vi "LEP_RV_MemorySettingsDlg.vi"(8 "error in (no error)":errorcluster, 10 "page sync rendezvous":T2, 11 "Close Event":refnum<user-event>) -> ()   [LabVIEW 2011]
doc: "This is the actual UI that the end user will see for configuring the build options."
uses:
  resource/dialog/PreferencesDialog/optionsFrame_EventData1.ctl
  resource/dialog/PreferencesDialog/optionsFrame_PageInitData.ctl
  <vilib>/Platform/EmbProject/Plugins/utilities/LEP_Utilities_GetSetProjectData_Variant.vi
panel:
  out "Tab Control":enum32{"Page 1", "Page 2"}(tab)
  in  "String":string
  in  "String 2":string
  in  "String 3":string
  in  "String 4":string
  in  "String 5":string
  in  "String 6":string
  in  "String 7":string
  in  "String 8":string
  in  "String 9":string
  in  "String 10":string
  in  "Boolean":bool
  in  "Boolean 2":bool
  in  "Boolean 3":bool
  in  "Boolean 4":bool
  in  "Boolean 5":bool
  in  "Boolean 6":bool
  in  "Boolean 7":bool
  in  "Boolean 8":bool
  in  "Boolean 9":bool
  in  "Boolean 10":bool
  in  "String 11":string
  in  "String 12":string
  in  "String 13":string
  in  "String 14":string
  in  "String 15":string
  in  "String 16":string
  in  "String 17":string
  in  "String 18":string
  in  "String 19":string
  in  "String 20":string
  in  "Boolean 11":bool
  in  "Boolean 12":bool
  in  "Boolean 13":bool
  in  "Boolean 14":bool
  in  "Boolean 15":bool
  in  "Boolean 16":bool
  in  "Boolean 17":bool
  in  "Boolean 18":bool
  in  "Boolean 19":bool
  in  "Boolean 20":bool
  in  "Ring 3":u16(ring) items=["<default>", "RAM1", "RAM2", "RAM3", "IRAM1", "IRAM2"]
  in  "Ring 2":u16(ring) items=["<default>", "RAM1", "RAM2", "RAM3", "IRAM1", "IRAM2"]
  in  "Ring":u16(ring) items=["<default>", "ROM1", "ROM2", "ROM3", "IROM1", "IROM2", "RAM1", "RAM2", "RAM3", "IRAM1", "IRAM2"]
  in  "Tree":string(tree)
  in  "Linker":path[](array[path])=[path ""]
  in  "Compiler":path[](array[path])=[path ""]
  out "Linker Flags":string
  out "Compiler Flags":string
  in  "ErrorFile":path
  in  "Extra LFlags":string
  in  "Extra CFlags":string
  in  "Debug Mode":u16(ring) items=["None", "Generate Debug Info", "On Chip", "On Chip (Release)"]
  in  "Generate C Function Calls":bool
  in  "Generate Integer Only":bool=TRUE
  in  "Show build warnings":bool
  in  "Build configuration":u16(ring) items=["Debug", "Release"]
  in  "Memory model":i32(ring) items=["Small", "Static"]
  in  "Use stack variables":bool
  in  "Generate serial only":bool
  in  "Generate guard code":bool
  in  "Page VI Init Data":T1
  in  "error msg format string":string="There was a problem applying the options from the %s category. The error message is \"%s.\""
  # "Build options"
  # "Debug options"
  # "Memory options"
  # "Run-time options"
  # "Read Only Memory Area"
  # "Default"
  # "Off-chip"
  # "Start"
  # "Size"
  # "Startup"
  # "ROM1:"
  # "ROM2:"
  # "ROM3:"
  # "On-chip"
  # "IROM1:"
  # "IROM2:"
  # "Read/Write Memory Area"
  # "Default"
  # "Off-chip"
  # "Start"
  # "Size"
  # "NoInit"
  # "RAM1:"
  # "RAM2:"
  # "RAM3:"
  # "On-chip"
  # "IRAM1:"
  # "IRAM2:"
  # "Memory Assignment"
  # "Code / Const:"
  # "Zero Initialized Data:"
  # "Other Data:"
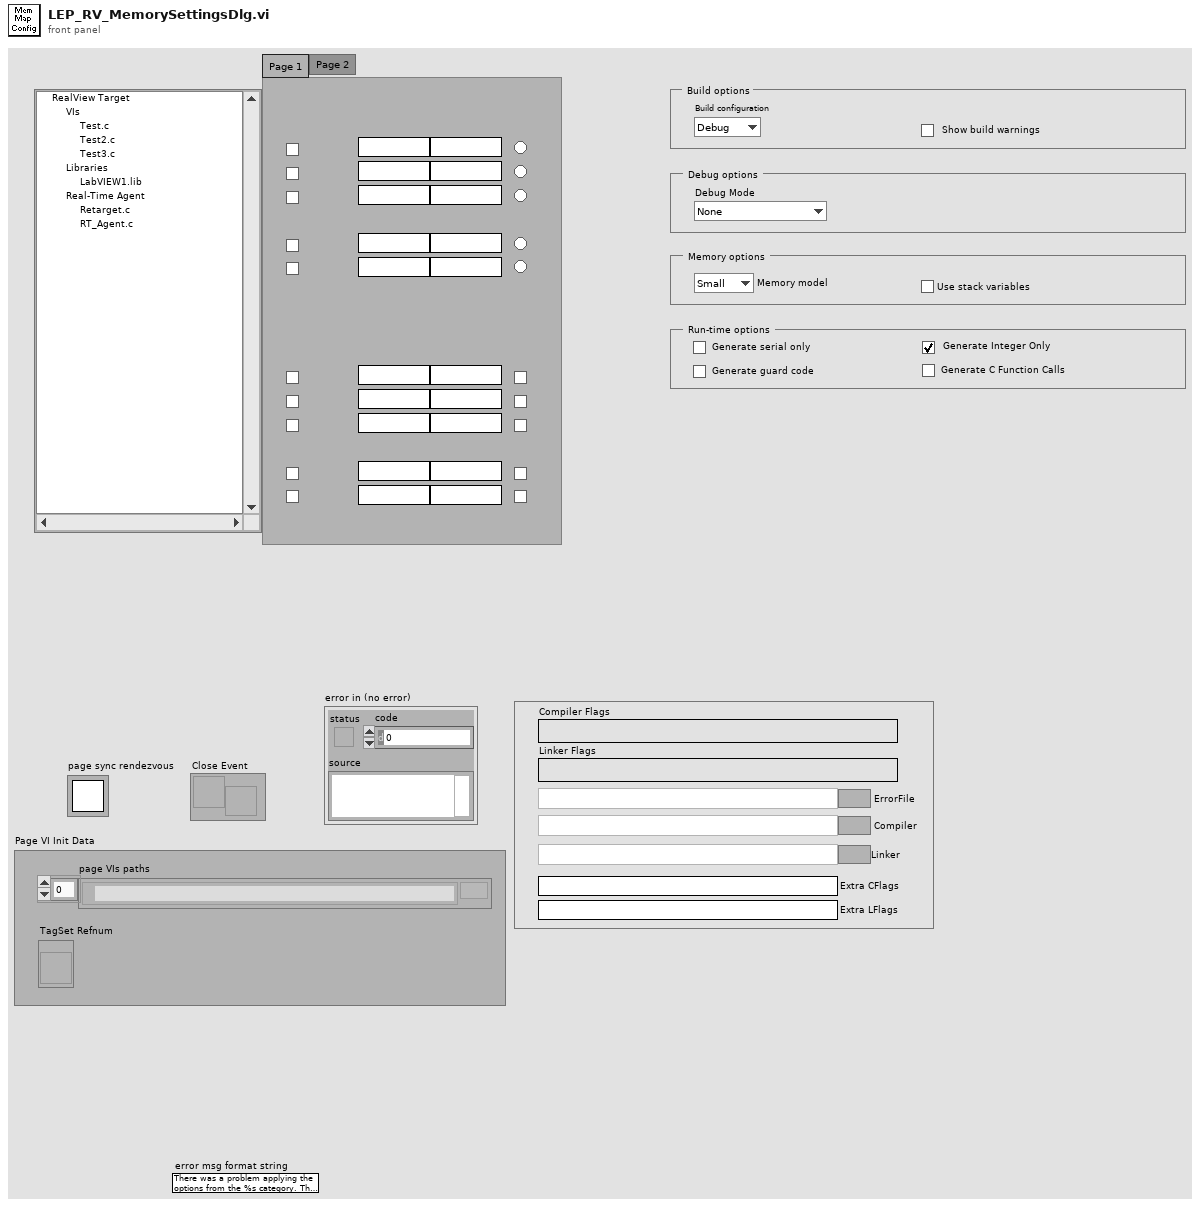
[diagram p1: front panel]
types:
  T1 = typedef "optionsFrame_PageInitData.ctl" = cluster{"page VIs paths":path[], "TagSet Refnum":refnum<vi>}
  T2 = typedef "Rendezvous RefNum" = refnum<k1>
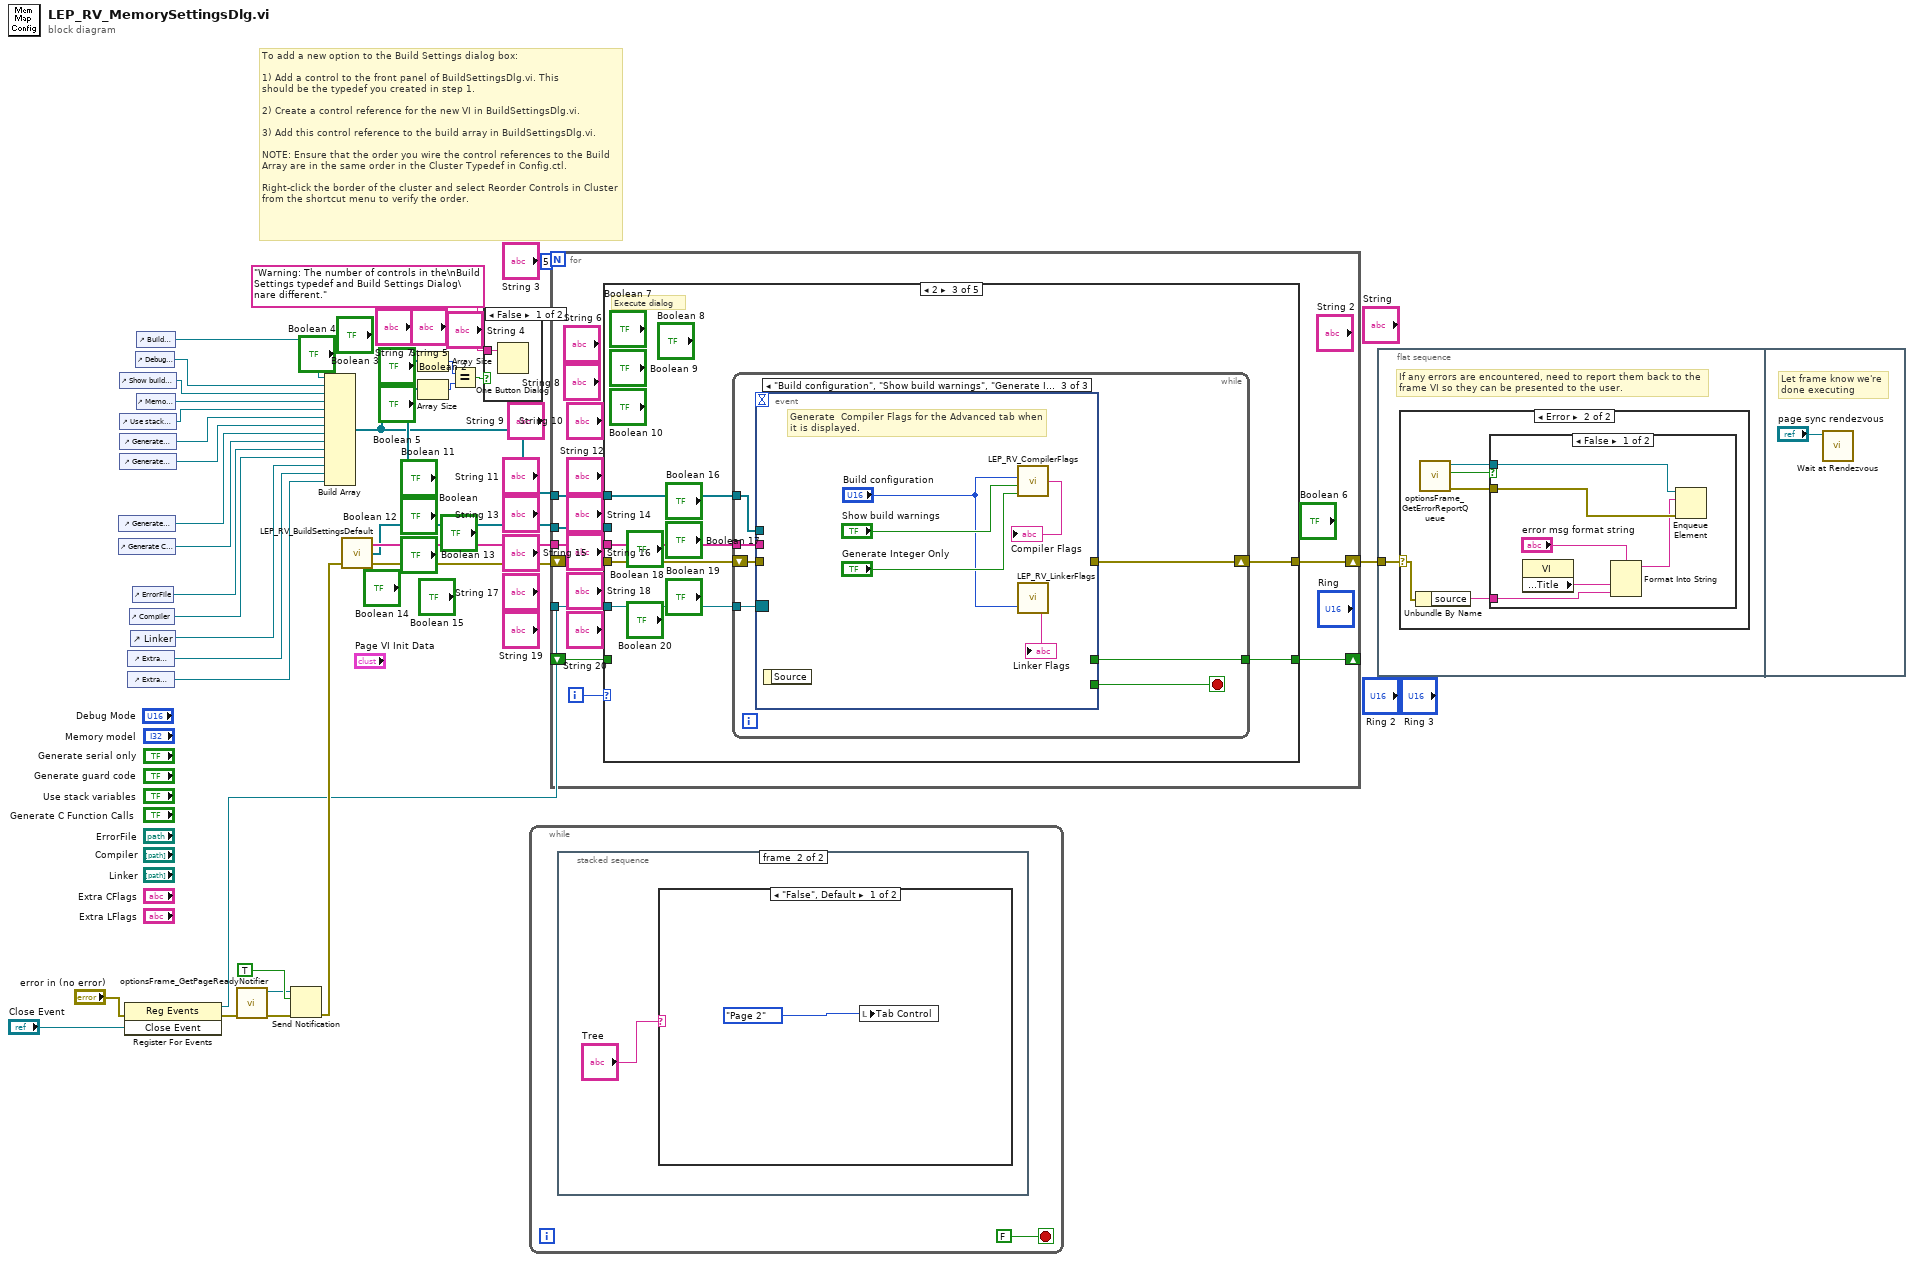
[diagram p0: block diagram]
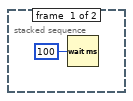
[diagram p2: hidden frame]
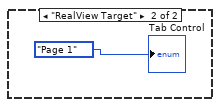
[diagram p3: hidden frame]
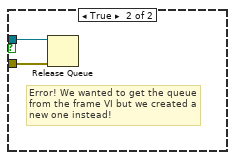
[diagram p5: hidden frame]
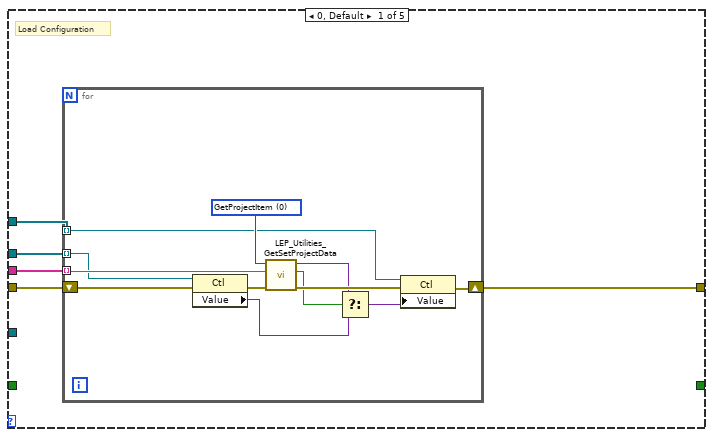
[diagram p7: hidden frame]
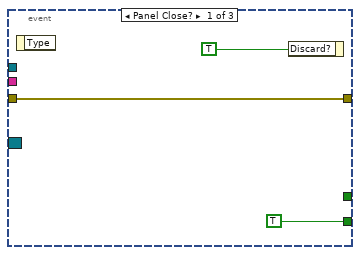
[diagram p9: hidden frame]
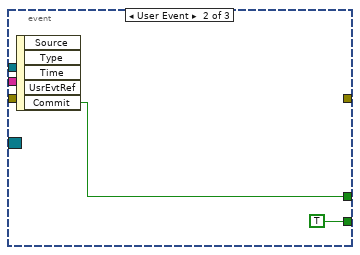
[diagram p10: hidden frame]
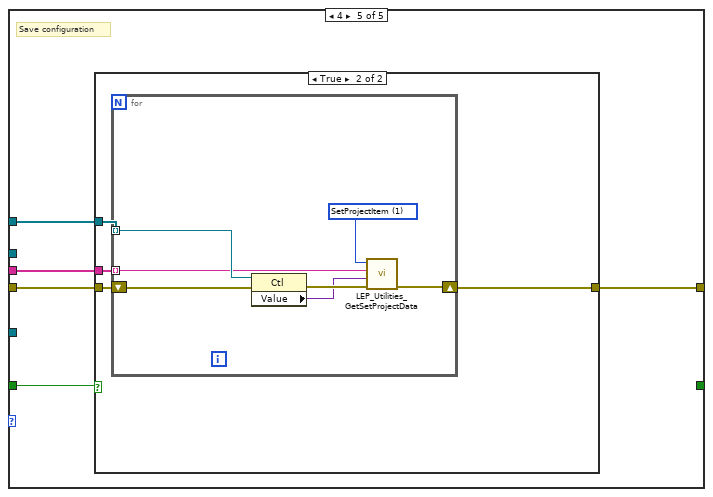
[diagram p12: hidden frame]
diagram:
  # "To add a new option to the Build Settings dialog box:\n\n1) Add a control to the front panel of BuildSettingsDlg.vi. This\nshould be the typedef you created in step 1.\n\n2) Create a control reference for the new VI in BuildSettingsDlg.vi.\n\n3) Add this control reference to the build array in BuildSettingsDlg.vi.\n\nNOTE: Ensure that the order you wire the control references to the Build Array are in the same order in the Cluster Typedef in Config.ctl.\n\nRight-click the border of the cluster and select Reorder Controls in Cluster from the shortcut menu to verify the order."
  n1 = control-ref of="Generate Integer Only"() -> (w23:refnum<vi>)
  n2 = control-ref of="Generate C Function Calls"() -> (w19:refnum<vi>)
  n3 = control-ref of="Show build warnings"() -> (w16:refnum<vi>)
  n4 = control-ref of="Use stack variables"() -> (w24:refnum<vi>)
  n5 = control-ref of="Generate serial only"() -> (w30:refnum<vi>)
  n6 = control-ref of="Generate guard code"() -> (w29:refnum<vi>)
  n7 = register-events(error in="error in (no error)", "Close Event") -> (reference out=w2:refnum<event-registration>, error out=w5:errorcluster)  [unwired: 1 in]
  n8 = control-ref of="Extra CFlags"() -> (w25:refnum<vi>)
  n9 = control-ref of="Extra LFlags"() -> (w26:refnum<vi>)
  n10 = control-ref of="Compiler"() -> (w22:refnum<vi>)
  n11 = control-ref of="Linker"() -> (w21:refnum<vi>)
  n12 = control-ref of="ErrorFile"() -> (w20:refnum<vi>)
  n13 = control-ref of="Debug Mode"() -> (w17:refnum<vi>)
  n14 = control-ref of="Build configuration"() -> (w18:refnum<vi>)
  n15 = control-ref of="Memory model"() -> (w31:refnum<vi>)
  n16 = call "optionsFrame_GetPageReadyNotifier.vi"("error in (no error)"=w5) -> ("error out"=w4:errorcluster, "notifier out"=w6:refnum<notifier>)  [unwired: 9 in]
  n17 = Send Notification(notification=TRUE, notifier=w6, error in (no error)=w4) -> (error out=w3:errorcluster)  [unwired: 1 out]
  n18 = Build Array(w18, w17, w16, w31, w24, w30, w29, w23, w19, w20, w22, w21, w25, w26) -> (w11:refnum<vi>[])
  n19 = call "LEP_RV_BuildSettingsDefault.vi"("error in (no error)"=w3) -> ("error out"=w28:errorcluster, "Default Values"=w12:refnum<vi>[], "Attribute Name"=w27:string[])  [unwired: 2 in]
  n20 = Array Size(array=w11) -> (size(s)=w14:i32)
  n21 = Array Size(array=w12) -> (size(s)=w15:i32)
  n22 = Equal?(x=w14, y=w15) -> (x = y?=w13:bool)
  n23 = case shown="False" w13 {
    tunnel: "Warning: The number of controls in the\nBuild Settings typedef and Build Settings Dialog\nare different." -> [w33 _]
    frame False {
      n24 = One Button Dialog(message=w33) -> ()  [unwired: 1 in, 1 out]
    }
    frame True {
    }
  }
  n25 = while {
    stop <- FALSE stop-if-true
    n26 = stacked-sequence {
      frame #0 {
        n27 = Wait (ms)(milliseconds to wait=u32 100) -> ()  [unwired: 1 out]
      }
      frame #1 {
        n28 = case shown="\"False\", Default" "Tree" {
          frame "False", Default {
            n29 = local write "Tab Control"(enum32{"Page 1", "Page 2"}."Page 2" ("Tab Control")) -> ()
          }
          frame "RealView Target" {
            "Tab Control" <- enum32{"Page 1", "Page 2"}."Page 1" ("Tab Control")
          }
        }
      }
    }
  }
  n30 = for {
    N: 5 -> [_]
    shift-right: [w45] -> w1
    shift-left: w28 -> [w46]
    shift-right: [w44] -> _
    shift-left: _ -> [w43]
    tunnel: w11 -> [w42]
    tunnel: w27 -> [w41]
    tunnel: w12 -> [w40]
    tunnel: w2 -> [w39]
    i -> [w47]
    n31 = case shown="2" w47 {
      tunnel: w46 -> [w51 w65 w71 w90 w94]
      tunnel: [w50 w65 w70 w90 w93] -> w45
      tunnel: [_ _ w69 w89 _] -> w44
      tunnel: w43 -> [_ _ _ w89 w95]
      tunnel: w42 -> [w52 _ w67 _ w91]
      tunnel: w41 -> [w49 _ w68 _ w92]
      tunnel: w40 -> [w48 _ _ _ _]
      tunnel: w39 -> [_ _ w66 _ _]
      frame 0, Default {
        # "Load Configuration"
        n32 = for {
          tunnel: w52 -> [w63] mode=indexing
          shift-right: [w61] -> w50
          shift-left: w51 -> [w59]
          tunnel: w49 -> [w60] mode=indexing
          tunnel: w48 -> [w57] mode=indexing
          w64 = u16 0 items=["GetProjectItem", "SetProjectItem"] ("Command")
          n33 = property class="Ctl"(reference=w57, error in=w59) -> (error out=w58:errorcluster, "Value"=w53:variant)  [unwired: 1 out]
          n34 = call-poly <vilib>:"LEP_Utilities_GetSetProjectData.vi"("error in"=w58, "ItemName"=w60, "Command"=w64) -> ("error out"=w62:errorcluster, "Found/Replaced?"=w54:bool, "Variant Out"=w55:variant)  [unwired: 6 in]
          n35 = Select(t=w55, s=w54, f=w53) -> (s? t:f=w56:variant)
          n36 = property class="Ctl"(reference=w63, error in=w62, "Value"=w56) -> (error out=w61:errorcluster)  [unwired: 1 out]
        }
      }
      frame 1 {
        # "Show dialog"
      }
      frame 2 {
        # "Execute dialog"
        n37 = while {
          shift-right: [w77] -> w70
          shift-left: w71 -> [w78]
          tunnel: [w76] -> w69
          tunnel: w68 -> [w74]
          tunnel: w67 -> [w73]
          tunnel: w66 -> [w72]
          stop <- w75 stop-if-true
          n38 = event shown="[2] \"Build configuration\", \"Show build warnings\", \"Generate Integer Only\": Value Change" {
            selector: w72 -> [_ _ _]
            dyn-events: _ -> [_ _ _]
            timeout: _ -> [_ _ _]
            tunnel: w78 -> [w80 _ _]
            tunnel: [w80 _ _] -> w77
            tunnel: [_ w82 _] -> w76
            tunnel: [TRUE TRUE ("Cancel") _] -> w75
            tunnel: w74 -> [_ _ _]
            tunnel: w73 -> [_ _ _]
            event Panel Close? {
              n39 = event-data() -> ()  [unwired: 1 in, 1 out]
              n40 = event-data("Discard?"=TRUE) -> ()  [unwired: 1 in, 1 out]
            }
            event User Event {
              n41 = event-data() -> ("Commit"=w82:bool)  [unwired: 1 in, 4 out]
            }
            event "Build configuration", "Show build warnings", "Generate Integer Only": Value Change {
              # "Generate  Compiler Flags for the Advanced tab when\nit is displayed."
              n42 = event-data() -> ()  [unwired: 1 in, 1 out]
              n43 = call "LEP_RV_CompilerFlags.vi"("Generate Integer Only"="Generate Integer Only", "Show compile warnings"="Show build warnings", "Build configuration"="Build configuration") -> ("CFlags"=→"Compiler Flags":string)  [unwired: 1 in]
              n44 = call "LEP_RV_LinkerFlags.vi"("Build configuration"="Build configuration") -> ("LFlags"=→"Linker Flags":string)  [unwired: 1 in]
            }
          }
        }
      }
      frame 3 {
        # "Close dialog"
      }
      frame 4 {
        # "Save configuration"
        n45 = case shown="True" w95 {
          tunnel: w94 -> [w96 w100]
          tunnel: [w96 w97] -> w93
          tunnel: w92 -> [_ w99]
          tunnel: w91 -> [_ w98]
          frame False {
          }
          frame True {
            n46 = for {
              shift-right: [w101] -> w97
              shift-left: w100 -> [w106]
              tunnel: w99 -> [w103] mode=indexing
              tunnel: w98 -> [w105] mode=indexing
              w107 = u16 1 items=["GetProjectItem", "SetProjectItem"] ("Command")
              n47 = property class="Ctl"(reference=w105, error in=w106) -> (error out=w104:errorcluster, "Value"=w102:variant)  [unwired: 1 out]
              n48 = call-poly <vilib>:"LEP_Utilities_GetSetProjectData.vi"("error in"=w104, "Variant In"=w102, "ItemName"=w103, "Command"=w107) -> ("error out"=w101:errorcluster)  [unwired: 5 in, 2 out]
            }
          }
        }
      }
    }
  }
  n49 = flat-sequence {
    tunnel: w1 -> [w108]
    frame #0 {
      # "If any errors are encountered, need to report them back to the \nframe VI so they can be presented to the user."
      n50 = case shown="Error" w108 {
        selector: w108 -> [_ w110]
        frame No Error {
        }
        frame Error {
          n51 = Unbundle By Name(w110) -> ("source"=w109:string)
          n52 = call "optionsFrame_GetErrorReportQueue.vi"() -> ("error out"=w111:errorcluster, "created new?"=w113:bool, "queue out"=w112:refnum<queue>)  [unwired: 9 in]
          n53 = case shown="False" w113 {
            tunnel: w112 -> [w119 w121]
            tunnel: w111 -> [w118 w120]
            tunnel: w109 -> [w115 _]
            frame False {
              n54 = property class="VI"() -> ("Front Panel.Title"=w116:string)  [unwired: 2 in, 2 out]
              n55 = Format Into String(format string="error msg format string", w116, w115) -> (resulting string=w114:string)  [unwired: 2 in, 1 out]
              n56 = Enqueue Element(queue=w119, element=w114, error in (no error)=w118) -> ()  [unwired: 1 in, 3 out]
            }
            frame True {
              # "Error! We wanted to get the queue\nfrom the frame VI but we created a\nnew one instead!"
              n57 = Release Queue(queue=w121, error in (no error)=w120) -> ()  [unwired: 1 in, 3 out]
            }
          }
        }
      }
    }
    frame #1 {
      # "Let frame know we're \ndone executing"
      n58 = call <vilib>:"Wait at Rendezvous.vi"("rendezvous"="page sync rendezvous") -> ()  [unwired: 4 in, 3 out]
    }
  }
